vi "Simple H5Aread (Variant).vi"(4 "Type":variant, 6 "error in (no error)":errorcluster, 8 "Name":string, 9 "HDF5 Ref":T1) -> (0 "error out":errorcluster, 2 "Value":variant, 3 "HDF5 Ref out":T1)   [LabVIEW 2017]
doc: "Reads a named attribute attached to the specified HDF5 object"
uses:
  <vilib>/UPVI/lvhdf5/library.llb/HDF5 Ref.ctl
panel:
  # "LVHDF5 Toolkit\nCopyright (c) 2005-2013 by Jason D. Sommerville\nCopyright (c) 2014 by UPVI, LLC.\n\nThis use and distribution of this file is governed by the terms found in \nLICENSE.txt distributed with this toolkit and installed at\n <user.lib>\\_lvhdf5\\LICENSE.txt"
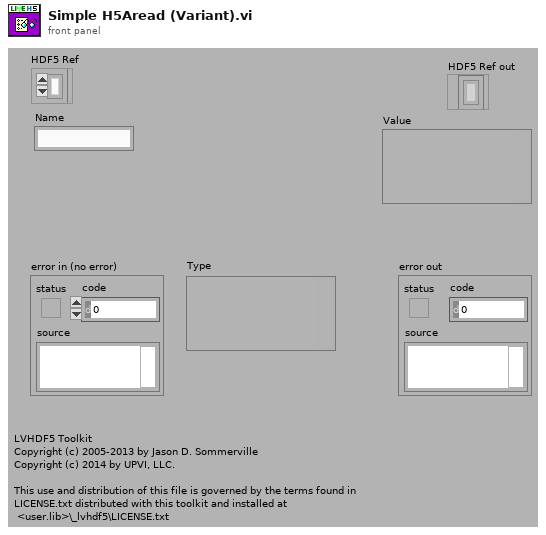
[diagram p1: front panel]
types:
  T1 = typedef "HDF5 Ref.ctl" = refnum<k1>
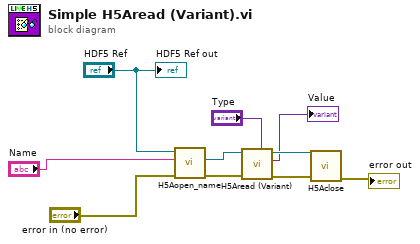
[diagram p0: block diagram]
diagram:
  n1 = call <vilib>:"H5Aopen_name.vi"("error in (no error)"="error in (no error)", "name"="Name", "HDF5 Ref"="HDF5 Ref") -> ("error out"=w7:errorcluster, "HDF5 Attr Ref"=w10:T1)  [unwired: 4 in, 1 out]
  n2 = call <vilib>:"H5Aread (Variant).vi"("Data"="Type", "error in (no error)"=w7, "HDF5 Attr Ref"=w10) -> ("error out"=w4:errorcluster, "Data out"=→"Value":variant, "HDF5 Attr Ref out"=w9:T1)  [unwired: 4 in]
  n3 = call <vilib>:"H5Aclose.vi"("error in (no error)"=w4, "HDF5 Dataset Ref"=w9) -> ("error out"=→"error out":errorcluster)  [unwired: 7 in]
  "HDF5 Ref out" <- "HDF5 Ref"
